vi "Setup High Frequency Clock Generation.vi"() -> ()   [LabVIEW 2013]
doc: "Setups the clock to a high frequency mode and then saves it to a known config slot."
uses:
  <instrlib>/Stanford Research CG635/Stanford Research CG635.lvlib
panel:
  in  "VISA resource name":refnum<visa-resource-name>
  in  "Q / Q  Level (0: ECL)":u16(ring) items=["ECL Levels (-1.00/-1.80 V)", "+7 dBm Levels (+0.50/-0.50 V)", "LVDS Levels (1.43/1.07 V)", "PECL 3.3 V Levels (2.30/1.50 V)", "PECL 5.0 V Levels (4.00/3.20 V)", ""]
  in  "CMOS Level (0: 1.2V)":u16(ring) items=["1.2 V", "1.8 V", "2.5 V", "3.3 V", "5.0 V"]
  in  "Unit (1:GHz)":u16(ring) items=["GHz", "MHz", "KHz", "Hz"]
  in  "Frequency (2.05)":dbl=2.05
  # "(c) 2014 National Instruments.  ALL RIGHTS RESERVED."
  # "For this example, the frequency is set to the max setting of 2.05 GHz. The \nnormal default value is 10 MHz."
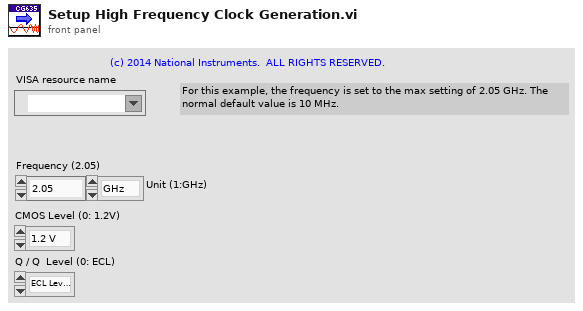
[diagram p1: front panel]
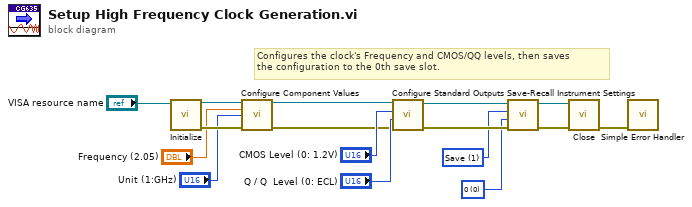
[diagram p0: block diagram]
diagram:
  w11 = u16 0 items=["0", "1", "2", "3", "4", "5", "6", "7"] ("Save Number (0)")
  w12 = u16 1 items=["Recall", "Save"] ("Recall or Save (0:Recall)")
  # "Configures the clock's Frequency and CMOS/QQ levels, then saves\nthe configuration to the 0th save slot."
  n1 = call <instrlib>:"Initialize.vi"("VISA resource name"="VISA resource name") -> ("error out"=w4:errorcluster, "VISA resource name out"=w6:refnum<visa-resource-name>)  [unwired: 9 in]
  n2 = call <instrlib>:"Configure Component Values.vi"("VISA resource name"=w6, "Frequency (10)"="Frequency (2.05)", "Unit (1:MHz)"="Unit (1:GHz)", "error in (no error)"=w4) -> ("VISA resource name out"=w5:refnum<visa-resource-name>, "error out"=w3:errorcluster)  [unwired: 10 in]
  n3 = call <instrlib>:"Configure Standard Outputs.vi"("error in (no error)"=w3, "Q / Q  Level (0: ECL)"="Q / Q  Level (0: ECL)", "CMOS Level (0: 1.2V)"="CMOS Level (0: 1.2V)", "VISA resource name"=w5) -> ("error out"=w13:errorcluster, "VISA resource name out"=w14:refnum<visa-resource-name>)  [unwired: 6 in]
  n4 = call <instrlib>:"Save-Recall Instrument Settings.vi"("error in (no error)"=w13, "Save Number (0)"=w11, "Recall or Save (0:Recall)"=w12, "VISA resource name"=w14) -> ("error out"=w9:errorcluster, "VISA resource name out"=w10:refnum<visa-resource-name>)  [unwired: 6 in]
  n5 = call <instrlib>:"Close.vi"("error in (no error)"=w9, "VISA resource name"=w10) -> ("error out"=w8:errorcluster)  [unwired: 9 in]
  n6 = call <vilib>:"Simple Error Handler.vi"("error in (no error)"=w8) -> ()  [unwired: 4 in, 5 out]
